vi "CloseChannel(SubVI).vi"(11 "VISA Refnum in":refnum<visa-resource-name>) -> ()   [LabVIEW 2022 SP3]
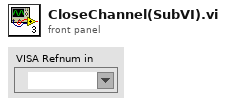
[diagram p1: front panel]
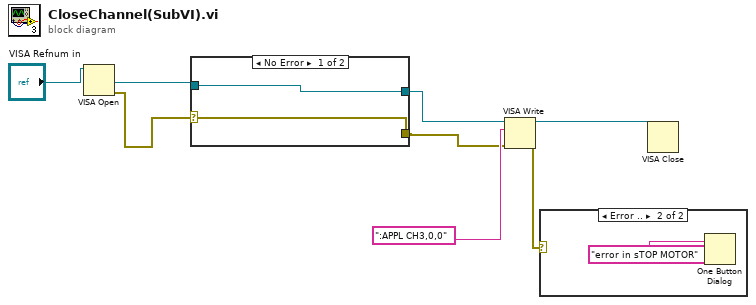
[diagram p0: block diagram]
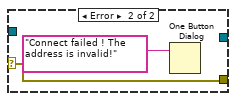
[diagram p2: hidden frame]
diagram:
  n1 = VISA Open(VISA resource name="VISA Refnum in") -> (VISA resource name=w2:refnum<visa-resource-name>, error out=w4:errorcluster)  [unwired: 4 in]
  n2 = case shown="No Error" w4 {
    selector: w4 -> [w9 w11]
    tunnel: w2 -> [w10 _]
    tunnel: [w10 _] -> w5
    tunnel: [w9 w11] -> w1
    frame No Error {
    }
    frame Error {
      n3 = One Button Dialog(message="Connect failed ! The address is invalid!") -> ()  [unwired: 1 in, 1 out]
    }
  }
  n4 = VISA Write(VISA resource name=w5, write buffer=":APPL CH3,0,0", error in (no error)=w1) -> (VISA resource name out=w6:refnum<visa-resource-name>, error out=w8:errorcluster)  [unwired: 1 out]
  n5 = case shown="Error .." w8 {
    frame No Error {
    }
    frame Error {
      n6 = One Button Dialog(message="error in sTOP MOTOR") -> ()  [unwired: 1 in, 1 out]
    }
  }
  n7 = VISA Close(VISA resource name=w6) -> ()  [unwired: 1 in, 1 out]
